vi "Unbox.vi"(10 "CustomeNode in":refnum<class "CustomeNode.lvclass">) -> (2 "data":i32)   [LabVIEW 2010, in "CustomeNode.lvclass"]
uses:
  CustomeNode.lvclass
  CustomeNode.lvclass/CustomeNode.ctl
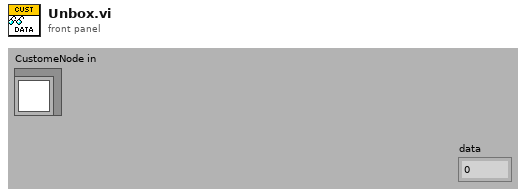
[diagram p1: front panel]
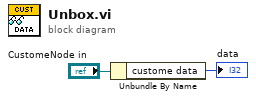
[diagram p0: block diagram]
diagram:
  n1 = Unbundle By Name("CustomeNode in") -> ("custome data"=→"data":i32)
